vi "ControlSub.vi"(0 "AxisForceSample":dbl[](array[numeric]), 1 "Command":dbl[](array[numeric]), 3 "Angel":bool[](array[boolean]), 4 "AngleSample":dbl[](array[numeric]), 5 "TorqueSample":dbl[](array[numeric]), 6 "Torque":bool[](array[boolean]), 7 "TempAnIn":dbl[](array[numeric]), 9 "ChannelSetArray":T1[](array[typedef]) {"Enable" items=["不使能", "使能"]; "Wave" items=["0指令", "正弦波", "方波", "三角波", "常值", "波形数据", "白噪声", "正弦扫频", "梯度加载", "VMIC"]; "ChannelType" items=["标准波形跟踪"=1, "扫频测试"=2, "消除多余力"=3, "梯度加载"=4, "载荷谱跟踪"=5, "模拟输入跟踪"=9]; "ChannelStatus" items=["通道关", "位置通道", "加载通道"]}, 12 "ControlPara":dbl[][](array[numeric])) -> (10 "diff syn out 2":dbl[](array[numeric]), 13 "syn out":dbl[](array[numeric]), 14 "ControlOutput":dbl[](array[numeric]), 15 "Forward":dbl[](array[numeric]), 17 "TempAnOut":dbl[](array[numeric]), 18 "control out":dbl[](array[numeric]), 19 "Commandout":dbl[](array[numeric]))   [LabVIEW 2014]
uses:
  ChannelCommand.ctl
  Control 1.ctl
  WaveType.ctl
  MoterEnable.ctl
panel:
  out "syn-angle":dbl[](array[numeric])
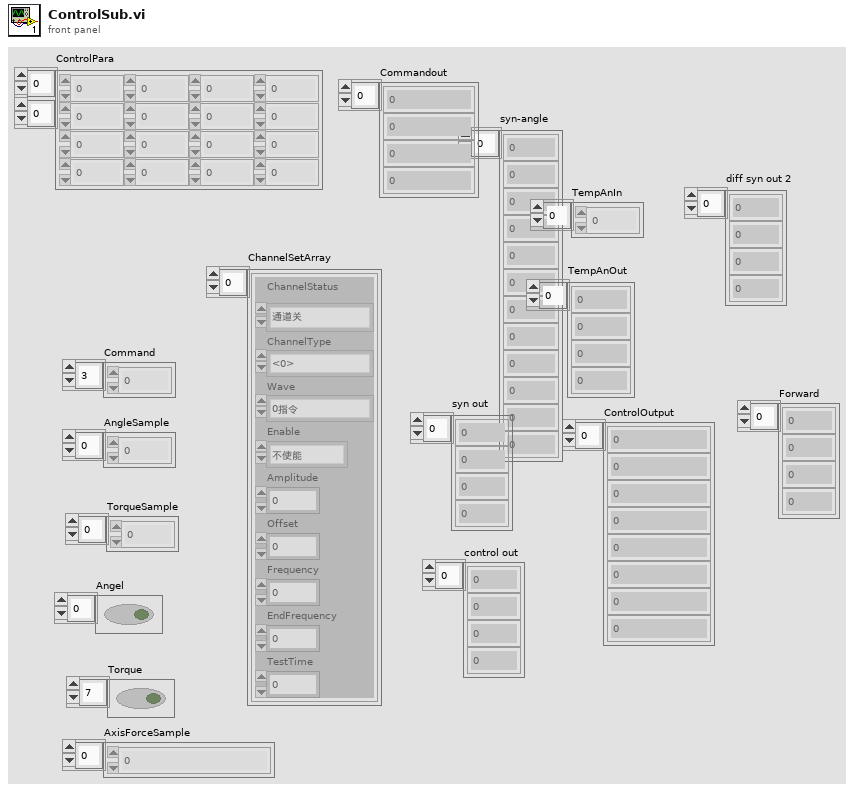
[diagram p1: front panel]
types:
  T1 = typedef "ChannelCommand.ctl" = cluster{"ChannelStatus":T2, "ChannelType":i32, "Wave":T3, "Enable":T4, "Amplitude":dbl, "Offset":dbl, "Frequency":dbl, "EndFrequency":dbl, "TestTime":dbl}
  T2 = typedef "Control 1.ctl" = i32
  T3 = typedef "WaveType.ctl" = i32
  T4 = typedef "MoterEnable.ctl" = u16
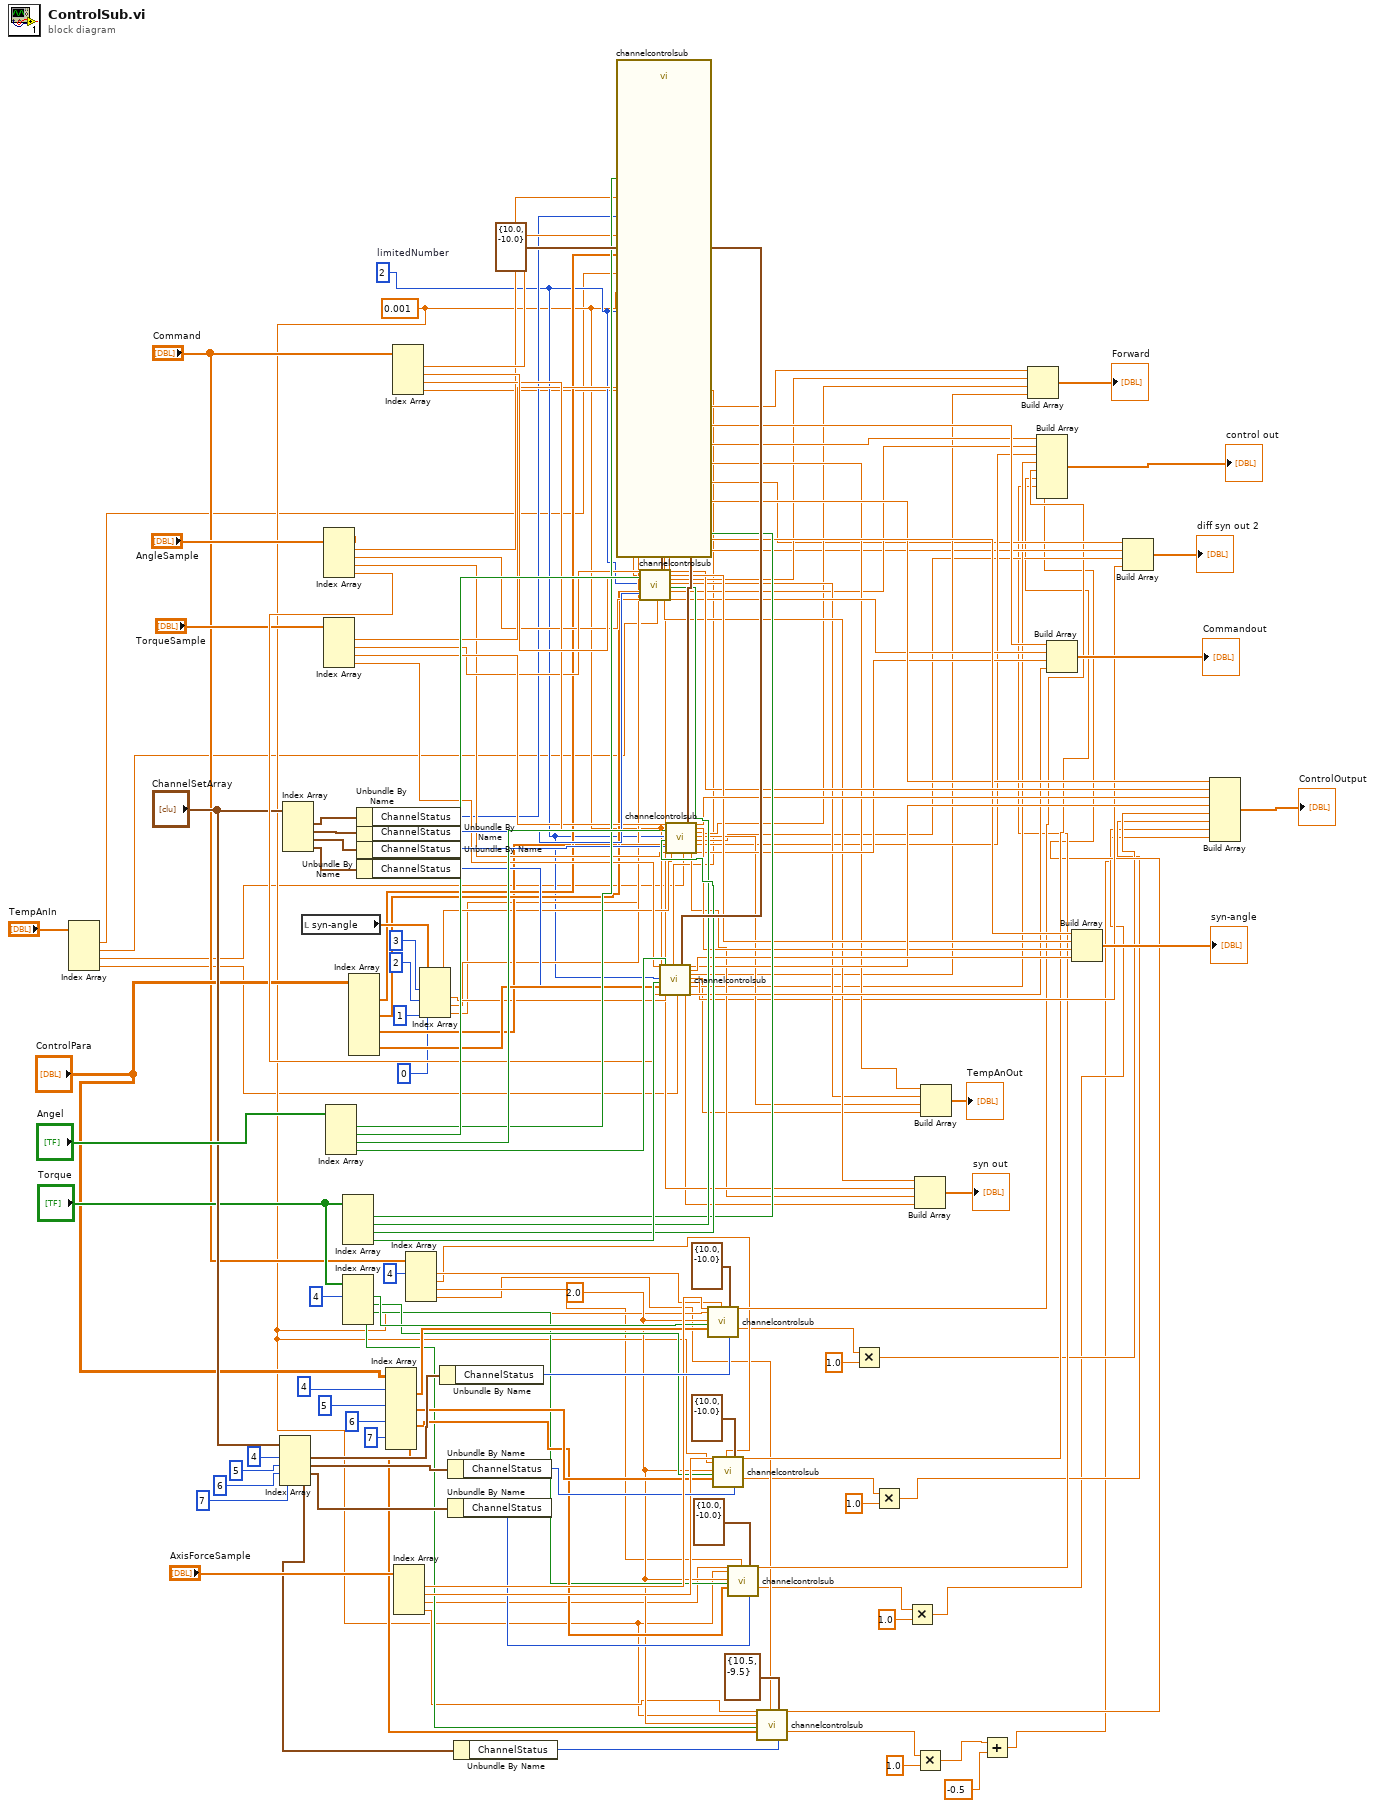
[diagram p0: block diagram]
diagram:
  w31 = 2.0 ("Limit Number")
  w26 = 0.001 ("dt")
  w89 = 2  # limitedNumber
  w147 = cluster{"output high":dbl, "output low":dbl} {"output high"=10.0, "output low"=-10.0} ("output range")
  n1 = Index Array(array="TempAnIn") -> (element #1=w4:dbl, element #2=w2:dbl, element #3=w3:dbl, element #4=w1:dbl)  [unwired: 4 in]
  n2 = Index Array(array="ChannelSetArray", index #1=4 ("索引"), index #2=5 ("索引"), index #3=6 ("索引"), index #4=7 ("索引")) -> (element #1=w61:T1, element #2=w47:T1, element #3=w38:T1, element #4=w30:T1)
  n3 = Index Array(array="ChannelSetArray") -> (element #1=w154:T1, element #2=w153:T1, element #3=w151:T1, element #4=w150:T1)  [unwired: 4 in]
  n4 = local read "syn-angle"() -> (w148:dbl[])
  n5 = Index Array(array="AngleSample") -> (element #1=w127:dbl, element #2=w126:dbl, element #3=w125:dbl, element #4=w76:dbl)  [unwired: 4 in]
  n6 = Index Array(array="TorqueSample") -> (element #1=w128:dbl, element #2=w129:dbl, element #3=w130:dbl, element #4=w131:dbl)  [unwired: 4 in]
  n7 = Index Array(array="Angel") -> (element #1=w139:bool, element #2=w140:bool, element #3=w141:bool, element #4=w142:bool)  [unwired: 4 in]
  n8 = Index Array(array="Torque") -> (element #1=w143:bool, element #2=w144:bool, element #3=w145:bool, element #4=w146:bool)  [unwired: 4 in]
  n9 = Index Array(array="Torque", index #1=4 ("索引")) -> (element #1=w56:bool, element #2=w40:bool, element #3=w39:bool, element #4=w32:bool)  [unwired: 3 in]
  n10 = Index Array(array="ControlPara") -> (element #1=w123:dbl[], element #2=w122:dbl[], element #3=w121:dbl[], element #4=w138:dbl[])  [unwired: 8 in]
  n11 = Unbundle By Name(w154) -> ("ChannelStatus"=w124:T2)
  n12 = Unbundle By Name(w153) -> ("ChannelStatus"=w135:T2)
  n13 = Unbundle By Name(w151) -> ("ChannelStatus"=w136:T2)
  n14 = Unbundle By Name(w150) -> ("ChannelStatus"=w137:T2)
  n15 = Index Array(array="ControlPara", index (row) #1=4 ("索引"), index (row) #2=5 ("索引 (行)"), index (row) #3=6 ("索引 (行)"), index (row) #4=7 ("索引 (行)")) -> (element #1=w53:dbl[], element #2=w44:dbl[], element #3=w41:dbl[], element #4=w35:dbl[])  [unwired: 4 in]
  n16 = Index Array(array="Command") -> (element #1=w134:dbl, element #2=w133:dbl, element #3=w132:dbl, element #4=w70:dbl)  [unwired: 4 in]
  n17 = Index Array(array="AxisForceSample") -> (element #1=w59:dbl, element #2=w45:dbl, element #3=w28:dbl, element #4=w27:dbl)  [unwired: 4 in]
  n18 = Index Array(array="Command", index #1=4 ("索引")) -> (element #1=w50:dbl, element #2=w21:dbl, element #3=w20:dbl, element #4=w19:dbl)  [unwired: 3 in]
  n19 = Index Array(array=w148, index #1=3 ("索引"), index #2=2 ("索引"), index #3=1 ("索引"), index #4=0 ("索引")) -> (element #1=w112:dbl, element #2=w111:dbl, element #3=w110:dbl, element #4=w109:dbl)
  n20 = Unbundle By Name(w61) -> ("ChannelStatus"=w67:T2)
  n21 = Unbundle By Name(w47) -> ("ChannelStatus"=w46:T2)
  n22 = Unbundle By Name(w38) -> ("ChannelStatus"=w37:T2)
  n23 = Unbundle By Name(w30) -> ("ChannelStatus"=w29:T2)
  n24 = call "channelcontrolsub.vi"("TorqueSample"=w128, "dt"=w26, "Limit Number"=w89, "Torque"=w143, "ControlPara"=w123, "AngleSample"=w127, "Angel"=w139, "syn-angel"=w110, "Command"=w134, "TempAngle"=w4, "output range"=w147, "ChannelStatus"=w124) -> ("syn out"=w101:dbl, "output"=w113:dbl, "syn-angle"=w114:dbl, "forward"=w87:dbl, "TempAngleOut"=w95:dbl, "diff syn out 2"=w82:dbl, "control out"=w92:dbl, "Commandout"=w107:dbl)  [unwired: 8 in]
  n25 = call "channelcontrolsub.vi"("TorqueSample"=w129, "dt"=w26, "Limit Number"=w89, "Torque"=w144, "ControlPara"=w122, "AngleSample"=w126, "Angel"=w140, "syn-angel"=w109, "Command"=w133, "TempAngle"=w2, "output range"=w147, "ChannelStatus"=w135) -> ("syn out"=w100:dbl, "output"=w115:dbl, "syn-angle"=w116:dbl, "forward"=w86:dbl, "TempAngleOut"=w96:dbl, "diff syn out 2"=w81:dbl, "control out"=w91:dbl, "Commandout"=w106:dbl)  [unwired: 8 in]
  n26 = call "channelcontrolsub.vi"("TorqueSample"=w131, "dt"=w26, "Limit Number"=w89, "Torque"=w146, "ControlPara"=w138, "AngleSample"=w76, "Angel"=w142, "syn-angel"=w111, "Command"=w70, "TempAngle"=w1, "output range"=w147, "ChannelStatus"=w137) -> ("syn out"=w98:dbl, "output"=w119:dbl, "syn-angle"=w120:dbl, "forward"=w84:dbl, "TempAngleOut"=w78:dbl, "diff syn out 2"=w80:dbl, "control out"=w79:dbl, "Commandout"=w104:dbl)  [unwired: 8 in]
  n27 = call "channelcontrolsub.vi"("TorqueSample"=w130, "dt"=w26, "Limit Number"=w89, "Torque"=w145, "ControlPara"=w121, "AngleSample"=w125, "Angel"=w141, "syn-angel"=w112, "Command"=w132, "TempAngle"=w3, "output range"=w147, "ChannelStatus"=w136) -> ("syn out"=w99:dbl, "output"=w117:dbl, "syn-angle"=w118:dbl, "forward"=w85:dbl, "TempAngleOut"=w97:dbl, "diff syn out 2"=w77:dbl, "control out"=w90:dbl, "Commandout"=w105:dbl)  [unwired: 8 in]
  n28 = call "channelcontrolsub.vi"("TorqueSample"=w59, "dt"=w26, "Limit Number"=w31, "Torque"=w56, "ControlPara"=w53, "Command"=w50, "output range"=cluster{"output high":dbl, "output low":dbl} {"output high"=10.0, "output low"=-10.0}, "ChannelStatus"=w67) -> ("output"=w25:dbl, "control out"=w18:dbl)  [unwired: 12 in, 6 out]
  n29 = call "channelcontrolsub.vi"("TorqueSample"=w45, "dt"=w26, "Limit Number"=w31, "Torque"=w40, "ControlPara"=w44, "Command"=w21, "output range"=cluster{"output high":dbl, "output low":dbl} {"output high"=10.0, "output low"=-10.0}, "ChannelStatus"=w46) -> ("output"=w24:dbl, "control out"=w15:dbl)  [unwired: 12 in, 6 out]
  n30 = call "channelcontrolsub.vi"("TorqueSample"=w28, "dt"=w26, "Limit Number"=w31, "Torque"=w39, "ControlPara"=w41, "Command"=w20, "output range"=cluster{"output high":dbl, "output low":dbl} {"output high"=10.0, "output low"=-10.0}, "ChannelStatus"=w37) -> ("output"=w23:dbl, "control out"=w11:dbl)  [unwired: 12 in, 6 out]
  n31 = call "channelcontrolsub.vi"("TorqueSample"=w27, "dt"=w26, "Limit Number"=w31, "Torque"=w32, "ControlPara"=w35, "Command"=w19, "output range"=cluster{"output high":dbl, "output low":dbl} {"output high"=10.5, "output low"=-9.5}, "ChannelStatus"=w29) -> ("output"=w22:dbl, "control out"=w8:dbl)  [unwired: 12 in, 6 out]
  n32 = Multiply(x=w18, y=1.0) -> (x*y=w16:dbl)
  n33 = Multiply(x=w15, y=1.0) -> (x*y=w14:dbl)
  n34 = Multiply(x=w11, y=1.0) -> (x*y=w10:dbl)
  n35 = Build Array(w101, w100, w99, w98) -> (→"syn out":dbl[])
  n36 = Multiply(x=w8, y=1.0) -> (x*y=w7:dbl)
  n37 = Build Array(w95, w96, w97, w78) -> (→"TempAnOut":dbl[])
  n38 = Add(x=w7, y=-0.5) -> (x+y=w5:dbl)
  n39 = Build Array(w87, w86, w85, w84) -> (→"Forward":dbl[])
  n40 = Build Array(w92, w91, w90, w79, w25, w24, w23, w22) -> (→"control out":dbl[])
  n41 = Build Array(w107, w106, w105, w104) -> (→"Commandout":dbl[])
  n42 = Build Array(w114, w116, w118, w120) -> (→"syn-angle":dbl[])
  n43 = Build Array(w82, w81, w77, w80) -> (→"diff syn out 2":dbl[])
  n44 = Build Array(w113, w115, w117, w119, w16, w14, w10, w5) -> (→"ControlOutput":dbl[])
